vi "Init Module.vi"(8 "error in":errorcluster, 11 "Singleton Module Admin in":refnum<class "Delacor_lib_QMH_Module Admin.lvclass">) -> (0 "error out":errorcluster, 2 "Acquisition Request Events":T1, 3 "Singleton Module Admin out":refnum<class "Delacor_lib_QMH_Module Admin.lvclass">)   [LabVIEW 2019, in "Acquisition.lvlib"]
doc: "Initialize the module by creating Broadcast Events, Request Events, and synchronization rendezvous.\n_____\nBased on Delacor QMH Project Template 4.0.0.47.\n_____\nBased on DQMH Project Template 6.1.0.94."
uses:
  Acquisition.lvlib
  <vilib>/Delacor/Delacor QMH/Libraries/Module Admin_class/Delacor_lib_QMH_Module Admin.lvclass
  Request Events--cluster.ctl
  Stop Argument--cluster.ctl
  Show Panel Argument--cluster.ctl
  Hide Panel Argument--cluster.ctl
  Get Module Execution Status Argument--cluster.ctl
  Show Diagram Argument--cluster.ctl
  Stop Acquiring Argument--cluster.ctl
  Wakeup Helper Loop Argument--cluster.ctl
  WiBCI16T_Data.ctl
  WiBCI16T_Status.ctl
  Reg_Map.ctl
  Acquisition Types.ctl
  Change Settings Argument--cluster.ctl
  Signal Type--enum.ctl
  Calibration Values--cluster.ctl
  Calibrate DAQ Argument--cluster.ctl
  Start Acquiring Argument--cluster.ctl
  Start Acquiring (Reply Payload)--cluster.ctl
  Command_TestData Argument--cluster.ctl
  Check WiFi AP Argument--cluster.ctl
  Command_NoiseData Argument--cluster.ctl
  Command_LiveData Argument--cluster.ctl
  Command_ImpedanceData Argument--cluster.ctl
  Command_GoToIdle Argument--cluster.ctl
  Soft Trigger Argument--cluster.ctl
  Start IMP Acquiring Argument--cluster.ctl
  Stop IMP acquiring Argument--cluster.ctl
  Start GND Loop acquiring Argument--cluster.ctl
  IMP data updated Argument--cluster.ctl
  IMP data updated (Reply Payload)--cluster.ctl
  Start CNV Acquiring Argument--cluster.ctl
  Start EOC Acquiring Argument--cluster.ctl
  Wake-up Helper Loop for Pkt Loss Calc Argument--cluster.ctl
  Stop Pkt Loss Calc Argument--cluster.ctl
  Update Packet ID Argument--cluster.ctl
  Calculate Packet Loss Argument--cluster.ctl
  Command_GndImpedanceData Argument--cluster.ctl
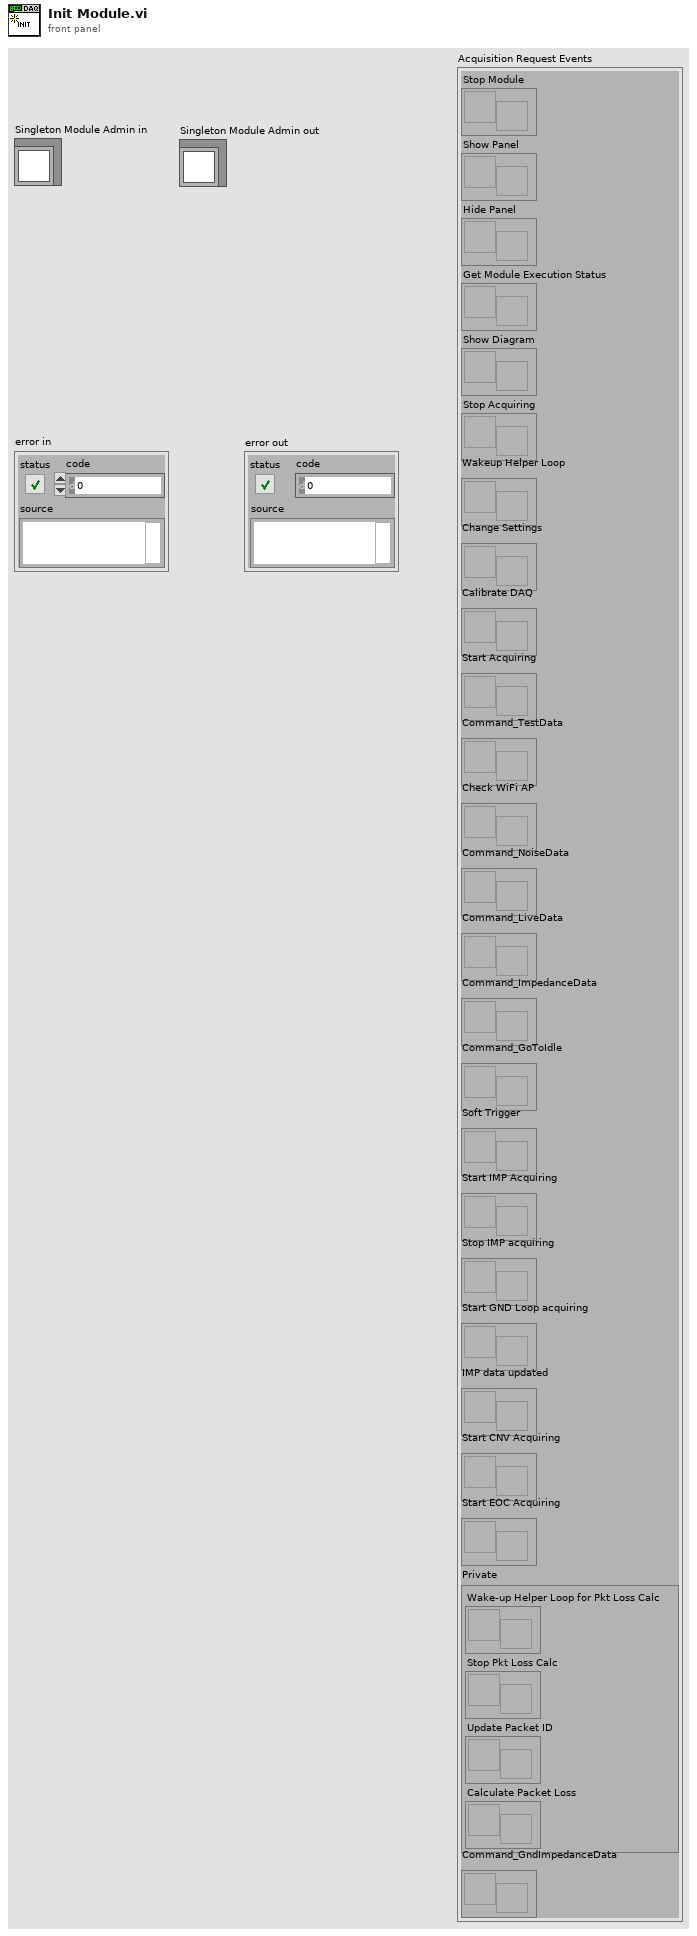
[diagram p1: front panel]
types:
  T1 = typedef "Acquisition.lvlib/Request Events--cluster.ctl" = cluster{"Stop Module":refnum<user-event>, "Show Panel":refnum<user-event>, "Hide Panel":refnum<user-event>, "Get Module Execution Status":refnum<user-event>, "Show Diagram":refnum<user-event>, "Stop Acquiring":refnum<user-event>, "Wakeup Helper Loop":refnum<user-event>, "Change Settings":refnum<user-event>, "Calibrate DAQ":refnum<user-event>, "Start Acquiring":refnum<user-event>, "Command_TestData":refnum<user-event>, "Check WiFi AP":refnum<user-event>, "Command_NoiseData":refnum<user-event>, "Command_LiveData":refnum<user-event>, "Command_ImpedanceData":refnum<user-event>, "Command_GoToIdle":refnum<user-event>, "Soft Trigger":refnum<user-event>, "Start IMP Acquiring":refnum<user-event>, "Stop IMP acquiring":refnum<user-event>, "Start GND Loop acquiring":refnum<user-event>, "IMP data updated":refnum<user-event>, "Start CNV Acquiring":refnum<user-event>, "Start EOC Acquiring":refnum<user-event>, "Private":cluster{"Wake-up Helper Loop for Pkt Loss Calc":refnum<user-event>, "Stop Pkt Loss Calc":refnum<user-event>, "Update Packet ID":refnum<user-event>, "Calculate Packet Loss":refnum<user-event>}, "Command_GndImpedanceData":refnum<user-event>}
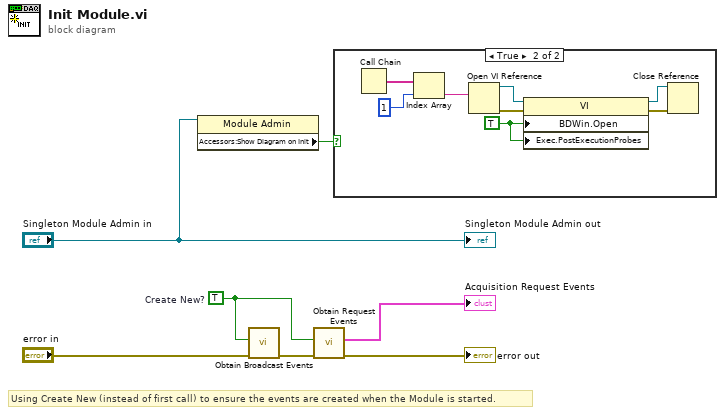
[diagram p0: block diagram]
diagram:
  w4 = TRUE  # Create New?
  # "Using Create New (instead of first call) to ensure the events are created when the Module is started."
  n1 = property class="Module Admin"(reference="Singleton Module Admin in") -> ("Accessors:Show Diagram on Init"=w2:bool)  [unwired: 1 in, 2 out]
  n2 = call "Obtain Broadcast Events.vi"("error in (no error)"="error in", "Create New? (F)"=w4) -> ("error out"=w7:errorcluster)  [unwired: 8 in, 1 out]
  n3 = call "Obtain Request Events.vi"("error in (no error)"=w7, "Create New? (F)"=w4) -> ("error out"=→"error out":errorcluster, "Acquisition Request Events"=→"Acquisition Request Events":T1)  [unwired: 8 in]
  n4 = case shown="True" w2 {
    frame False {
    }
    frame True {
      w11 = TRUE ("Block Diagram Window:Open")
      n5 = Call Chain() -> (call chain=w15:string[])
      n6 = Index Array(array=w15, index=1) -> (element=w8:string)
      n7 = Open VI Reference(vi path=w8) -> (vi reference=w12:refnum<vi>, error out=w13:errorcluster)  [unwired: 5 in]
      n8 = property class="VI"(reference=w12, error in=w13, "BDWin.Open"=w11, "Exec.PostExecutionProbes"=w11) -> (reference out=w9:refnum<vi>, error out=w10:errorcluster)
      n9 = Close Reference(reference=w9, error in (no error)=w10) -> ()  [unwired: 1 out]
    }
  }
  "Singleton Module Admin out" <- "Singleton Module Admin in"
